vi "SLSC Convert EDS Command to Tree Control Item.vi"(11 "command":T1) -> (2 "Glyph":i32, 3 "Child Text":string[](array[string]))   [LabVIEW 2017, in "SLSC Tree Control.lvlib"]
doc: "Convert the EDS property datatype to a Tree Control Child Text."
uses:
  SLSC Tree Control.lvlib
  Ctrl/command.ctl
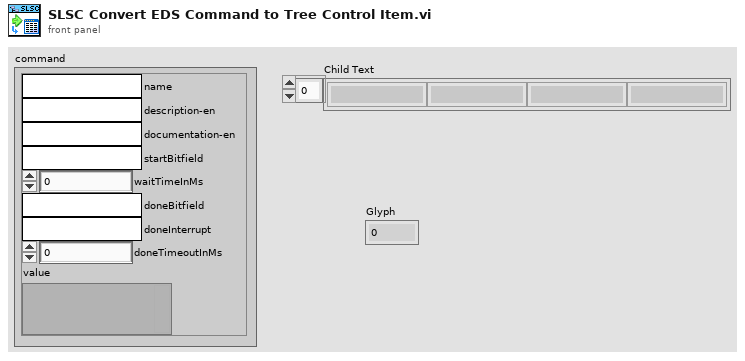
[diagram p1: front panel]
types:
  T1 = typedef "command.ctl" = cluster{"name":string, "description-en":string, "documentation-en":string, "startBitfield":string, "waitTimeInMs":i32, "doneBitfield":string, "doneInterrupt":string, "doneTimeoutInMs":i32, "value":variant}
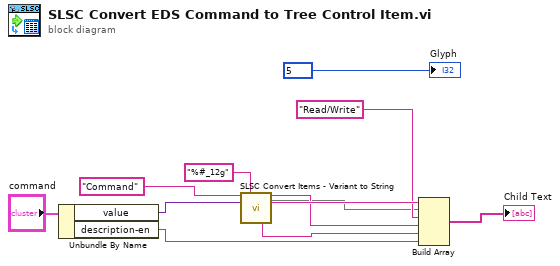
[diagram p0: block diagram]
diagram:
  n1 = Unbundle By Name("command") -> ("value"=w10:variant, "description-en"=w1:string)
  n2 = call "SLSC Convert Items - Variant to String.vi"("dataType"="Command", "format string"="%#_12g", "value"=w10) -> (3:w2, "Output data type"=w6:string, "string offline data value"=w7:string, "data_range"=w8:string)  [unwired: 7 in, 2 out]
  n3 = Build Array(w7, w2, "Read/Write" ("element"), w6, w8, w1) -> (→"Child Text":string[])
  "Glyph" <- 5
